vi "Event Teardown.vi"(11 "jettl Queue Actor in":refnum<class "jettl Queue Actor.lvclass">) -> (3 "jettl Queue Actor out":refnum<class "jettl Queue Actor.lvclass">)   [LabVIEW 2021, in "jettl.lvlib" / "jettl Queue Actor.lvlib" / "jettl Queue Actor.lvclass"]
uses:
  jettl Queue Actor.lvclass
  jettl Queue Actor.lvclass/jettl Queue Actor.ctl
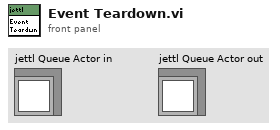
[diagram p1: front panel]
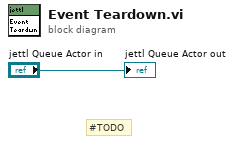
[diagram p0: block diagram]
diagram:
  # "#TODO"
  "jettl Queue Actor out" <- "jettl Queue Actor in"
